vi "Maintain Heading.vi"(8 "PID gains":T1={"proportional gain (Kc)"=1.0, "integral time (Ti, min)"=0.01, "derivative time (Td, min)"=0.0} {"derivative time (Td, min)" format="%.3f"; "integral time (Ti, min)" format="%.3f"; "proportional gain (Kc)" format="%.3f"}, 9 "NavX Yaw":dbl, 10 "Raw Driver Joystick X2":dbl) -> (3 "Driver Joystick X2":dbl)   [LabVIEW 2014]
uses:
  <vilib>/Rock Robotics/WPI/DriverStation/WPI_DriverStationRobotMode2.ctl
  Begin/Global Variables.vi
  <vilib>/addons/control/pid/pid.llb/PID (DBL).vi
  <vilib>/addons/control/pid/NI_PID_pid.lvlib
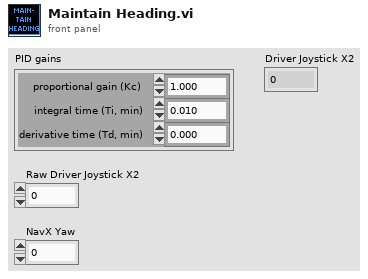
[diagram p1: front panel]
types:
  T1 = cluster{"proportional gain (Kc)":dbl, "integral time (Ti, min)":dbl, "derivative time (Td, min)":dbl}
  T2 = typedef "WPI_DriverStationRobotMode2.ctl" = enum16{"Autonomous Disabled", "Autonomous Enabled", "Teleop Disabled", "Teleop Enabled", "Disconnected", "Finish", "Test Disabled", "Test Enabled", "Emergency Stopped"}
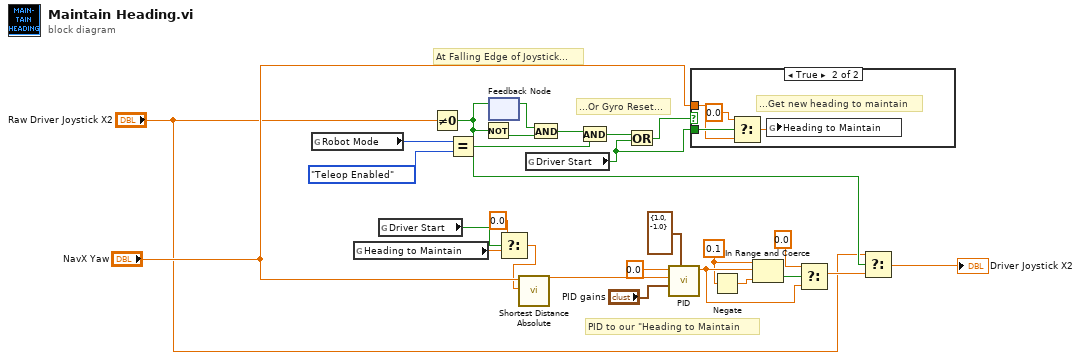
[diagram p0: block diagram]
diagram:
  w14 = 0.1 ("Value to Deadband (default of 0.1)")
  # "PID to our \"Heading to Maintain"
  # "...Or Gyro Reset..."
  # "At Falling Edge of Joystick..."
  n1 = global read "Global Variables.vi" "Robot Mode"() -> (w3:T2)
  n2 = global read "Global Variables.vi" "Heading to Maintain"() -> (w4:dbl)
  n3 = global read "Global Variables.vi" "Driver Start"() -> (w6:bool)
  n4 = Not Equal To 0?(x="Raw Driver Joystick X2") -> (x != 0?=w2:bool)
  n5 = Equal?(x=w3, y=WPI_DriverStationRobotMode2."Teleop Enabled") -> (x = y?=w19:bool)
  n6 = Not(x=w2) -> (.not. x?=w21:bool)
  n7 = feedback #1() -> (w20:bool)  [unwired: 1 in]
  n8 = feedback-in #1(w2) -> ()
  n9 = Select(t=0.0, s=w6, f=w4) -> (s? t:f=w5:dbl)
  n10 = call "Shortest Distance Absolute.vi"("current"=w5, "target"="NavX Yaw") -> ("shortest angle"=w10:dbl)  [unwired: 9 in]
  n11 = global read "Global Variables.vi" "Driver Start"() -> (w24:bool)
  n12 = And(x=w20, y=w21) -> (x .and. y?=w17:bool)
  n13 = And(x=w17, y=w19) -> (x .and. y?=w22:bool)
  n14 = Or(x=w22, y=w24) -> (x .or. y?=w23:bool)
  n15 = call-poly <vilib>:"PID.vi"("output range"=cluster{"output high":dbl, "output low":dbl} {"output high"=1.0, "output low"=-1.0}, "PID gains"="PID gains", "process variable"=w10, "setpoint"=0.0) -> ("output"=w16:dbl)  [unwired: 6 in, 1 out]
  n16 = case shown="True" w23 {
    tunnel: w24 -> [_ w31]
    tunnel: "NavX Yaw" -> [_ w28]
    frame False {
    }
    frame True {
      # "...Get new heading to maintain"
      n17 = Select(t=0.0, s=w31, f=w28) -> (s? t:f=w29:dbl)
      n18 = global write "Global Variables.vi" "Heading to Maintain"(w29) -> ()
    }
  }
  n19 = Negate(x=w14) -> (-x=w15:dbl)
  n20 = In Range and Coerce(upper limit=w14, x=w16, lower limit=w15) -> (In Range?=w13:bool)  [unwired: 1 out]
  n21 = Select(t=0.0, s=w13, f=w16) -> (s? t:f=w25:dbl)
  n22 = Select(t="Raw Driver Joystick X2", s=w2, f=w25) -> (s? t:f=→"Driver Joystick X2":dbl)
